vi "MRB_auto_ctrl_with_PTMR3.vi"(4 "ref_reinit":refnum<vi>, 6 "ref_O_set":refnum<vi>, 7 "array_value_in":dbl[](array[numeric]), 9 "P_set":dbl=0.5 caption="Set Point" format="%#_13g", 10 "enable_auto_ctrl":bool caption="Auto Control") -> (0 "O_new":dbl format="%.3f", 1 "auto_ctrl_status":u32(colorbox) caption="Status", 3 "P":dbl=1.1 format="%.2f", 5 "array_value_out":dbl[](array[numeric]))   [LabVIEW 2019]
doc: "This example demonstrates how to simulate a general PID controller."
uses:
  <vilib>/Analysis/baseanly.llb/Mean (DBL).vi
  MccHat/MccHat_Global.vi
  <vilib>/addons/control/pid/pid.llb/PID (DBL).vi
  <vilib>/addons/control/pid/NI_PID_pid.lvlib
  <vilib>/Analysis/NI_AALBase.lvlib
panel:
  in  "sp_step":dbl=0.1 format="%#_13g"
  in  "sp_nominal":dbl=10.0
  in  "sp_max":dbl=70.0
  in  "sp_min":dbl=5.0
  in  "n_avg":u8=3
  out "MV":dbl format="%.1f"
  in  "P_max":dbl=999.0 format="%.1f"
  in  "P_min":dbl=-0.4 format="%.1f"
  out "PID Range":cluster{"High":dbl, "Low":dbl}={"High"=20.0, "Low"=-20.0} {"Low" format="%.1f"; "High" format="%.1f"}
  in  "PID gains":T1={"proportional gain (Kc)"=-10.0, "integral time (Ti, min)"=0.2, "derivative time (Td, min)"=0.08} {"derivative time (Td, min)" format="%.4f"; "integral time (Ti, min)" format="%.4f"; "proportional gain (Kc)" format="%.3f"}
  # "psi"
  # "psi"
  # "psi"
  # "psig"
  # "K_c = dO/dP = -1/0.1 = -10.0\nT_i = 1.0 \nT_d = 0.1"
  # "L/m"
  # "L/m"
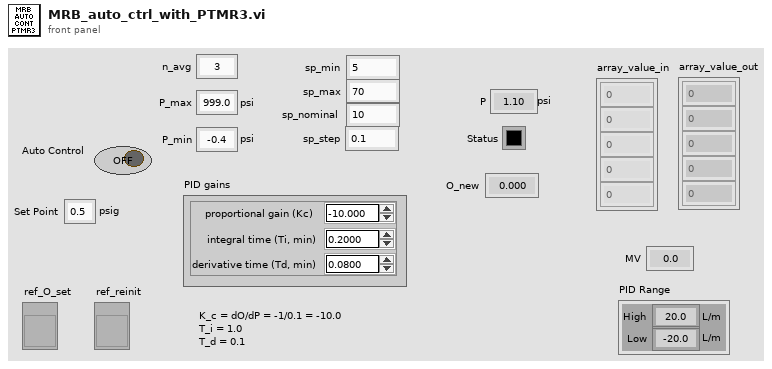
[diagram p1: front panel]
types:
  T1 = cluster{"proportional gain (Kc)":dbl, "integral time (Ti, min)":dbl, "derivative time (Td, min)":dbl}
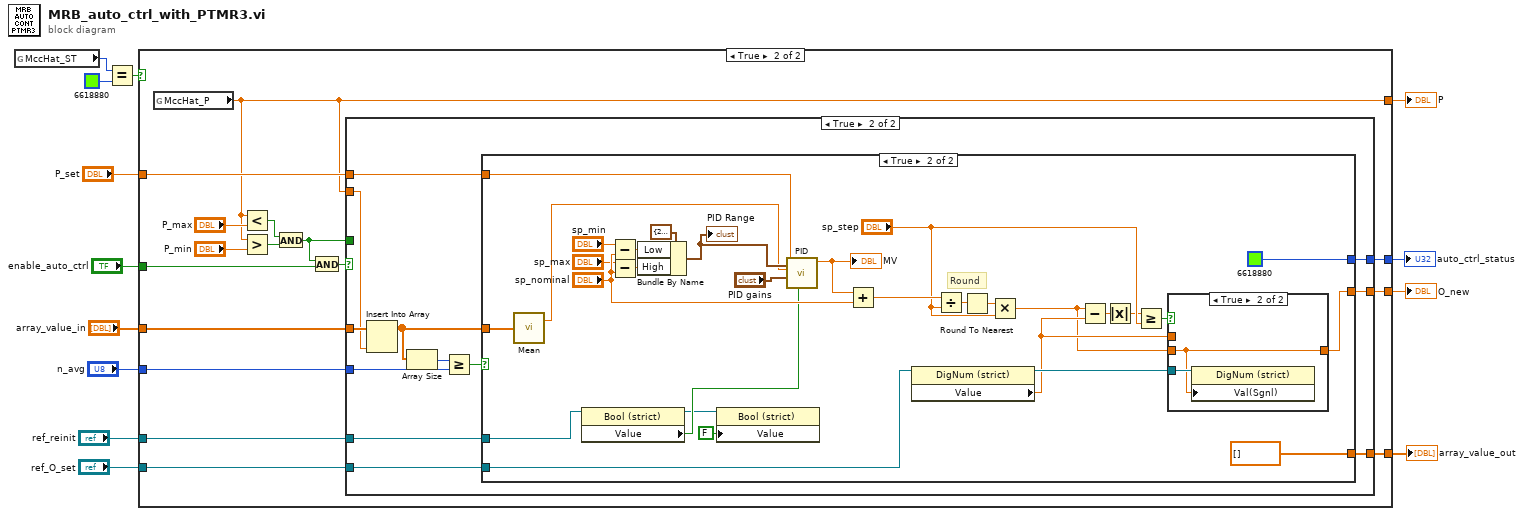
[diagram p0: block diagram]
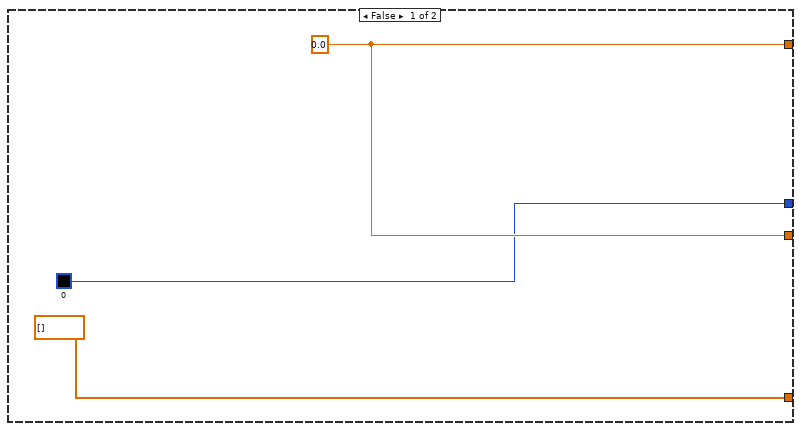
[diagram p2: hidden frame]
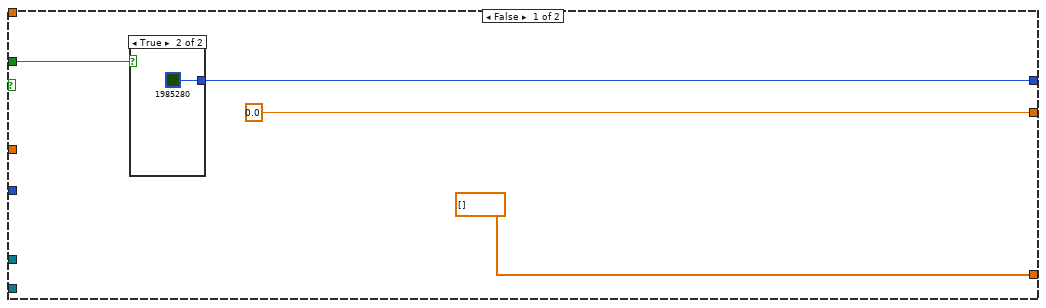
[diagram p3: hidden frame]
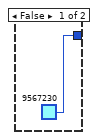
[diagram p4: hidden frame]
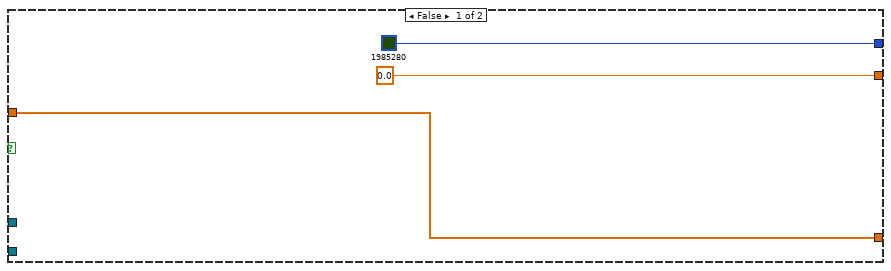
[diagram p5: hidden frame]
diagram:
  n1 = global read "MccHat_Global.vi" "MccHat_ST"() -> (w1:u32)
  n2 = Equal?(x=w1, y=u32 6618880 ("MG_ST")) -> (x = y?=w2:bool)
  n3 = case shown="True" w2 {
    tunnel: [w16 w32] -> w13
    tunnel: [u32 0 ("alarm_status") w31] -> w12
    tunnel: "P_set" -> [_ w21]
    tunnel: "enable_auto_ctrl" -> [_ w26]
    tunnel: [w16 w17] -> w9
    tunnel: "ref_O_set" -> [_ w28]
    tunnel: "ref_reinit" -> [_ w22]
    tunnel: "array_value_in" -> [_ w20]
    tunnel: "n_avg" -> [_ w19]
    tunnel: [dbl[] [] ("f") w18] -> w4
    frame False {
      w16 = 0.0 ("Value")
    }
    frame True {
      n4 = global read "MccHat_Global.vi" "MccHat_P"() -> (w17:dbl)
      n5 = Less?(x=w17, y="P_max") -> (x < y?=w24:bool)
      n6 = Greater?(x=w17, y="P_min") -> (0:w25:bool)
      n7 = And(x=w24, y=w25) -> (x .and. y?=w23:bool)
      n8 = And(x=w23, y=w26) -> (x .and. y?=w27:bool)
      n9 = case shown="True" w27 {
        tunnel: [0.0 ("F_O_new") w48] -> w32
        tunnel: [w34 w50] -> w31
        tunnel: w21 -> [_ w47]
        tunnel: w17 -> [_ w44]
        tunnel: w28 -> [_ w49]
        tunnel: w23 -> [w35 _]
        tunnel: w22 -> [_ w46]
        tunnel: w20 -> [_ w45]
        tunnel: w19 -> [_ w42]
        tunnel: [dbl[] [] ("f") w39] -> w18
        frame False {
          n10 = case shown="True" w35 {
            tunnel: [u32 9567230 ("alarm_status") u32 1985280 ("alarm_status")] -> w34
            frame False {
            }
            frame True {
            }
          }
        }
        frame True {
          n11 = Insert Into Array(array=w45, new element=w44) -> (w40:dbl[])  [unwired: 1 in]
          n12 = Array Size(array=w40) -> (size(s)=w43:i32)
          n13 = Greater Or Equal?(x=w43, y=w42) -> (x >= y?=w41:bool)
          n14 = case shown="True" w41 {
            tunnel: [u32 1985280 ("alarm_status") u32 6618880 ("alarm_status")] -> w50
            tunnel: w49 -> [_ w82]
            tunnel: [0.0 ("F_new") w81] -> w48
            tunnel: w47 -> [_ w79]
            tunnel: w46 -> [_ w77]
            tunnel: w40 -> [w51 w66]
            tunnel: [w51 dbl[] [] ("f")] -> w39
            frame False {
            }
            frame True {
              # "Round"
              n15 = call-poly <vilib>:"Mean.vi"("X"=w66) -> ("mean"=w65:dbl)  [unwired: 1 out]
              n16 = property class="Bool (strict)"(reference=w77) -> (reference out=w75:refnum<vi>, "Value"=w76:bool)  [unwired: 1 in, 1 out]
              n17 = Subtract(x="sp_min", y="sp_nominal") -> (x-y=w71:dbl)
              n18 = Subtract(x="sp_max", y="sp_nominal") -> (x-y=w72:dbl)
              n19 = Bundle By Name(cluster=cluster{"High":dbl, "Low":dbl} {"High"=20.0, "Low"=-20.0} ("PID Range"), "Low"=w71, "High"=w72) -> (w67:cluster{"High":dbl, "Low":dbl})
              "PID Range" <- w67
              n20 = property class="Bool (strict)"(reference=w75, "Value"=FALSE) -> ()  [unwired: 1 in, 2 out]
              n21 = call-poly <vilib>:"PID.vi"("reinitialize? (F)"=w76, "output range"=w67, "PID gains"="PID gains", "process variable"=w65, "setpoint"=w79) -> ("output"=w78:dbl)  [unwired: 5 in, 1 out]
              "MV" <- w78
              n22 = Add(x=w78, y="sp_nominal") -> (x+y=w61:dbl)
              n23 = property class="DigNum (strict)"(reference=w82) -> ("Value"=w63:dbl)  [unwired: 1 in, 2 out]
              n24 = Divide(x=w61, y="sp_step") -> (x/y=w58:dbl)
              n25 = Round To Nearest(number=w58) -> (nearest integer value=w59:dbl)
              n26 = Multiply(x=w59, y="sp_step") -> (x*y=w62:dbl)
              n27 = Subtract(x=w62, y=w63) -> (x-y=w55:dbl)
              n28 = Absolute Value(x=w55) -> (abs(x)=w56:dbl)
              n29 = Greater Or Equal?(x=w56, y="sp_step") -> (x >= y?=w57:bool)
              n30 = case shown="True" w57 {
                tunnel: w82 -> [_ w85]
                tunnel: w62 -> [_ w84]
                tunnel: [w83 w84] -> w81
                tunnel: w63 -> [w83 _]
                frame False {
                }
                frame True {
                  n31 = property class="DigNum (strict)"(reference=w85, "Val(Sgnl)"=w84) -> ()  [unwired: 1 in, 2 out]
                }
              }
            }
          }
        }
      }
    }
  }
  "O_new" <- w13
  "auto_ctrl_status" <- w12
  "P" <- w9
  "array_value_out" <- w4
